vi "Get Local Framework Fields.vi"(8 "error in":errorcluster) -> (0 "error out":errorcluster, 3 "ATS Framework Fields out":T1)   [LabVIEW 2022 SP3]
uses:
  Arcadia/Common/Framework/ATS Framework Fields.ctl
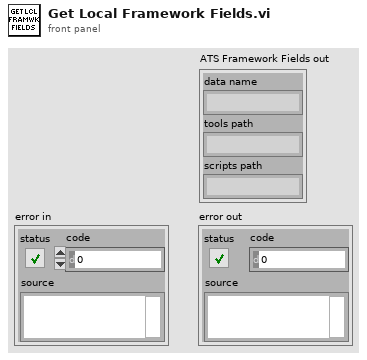
[diagram p1: front panel]
types:
  T1 = typedef "ATS Framework Fields.ctl" = cluster{"data name":string, "tools path":string, "scripts path":string}
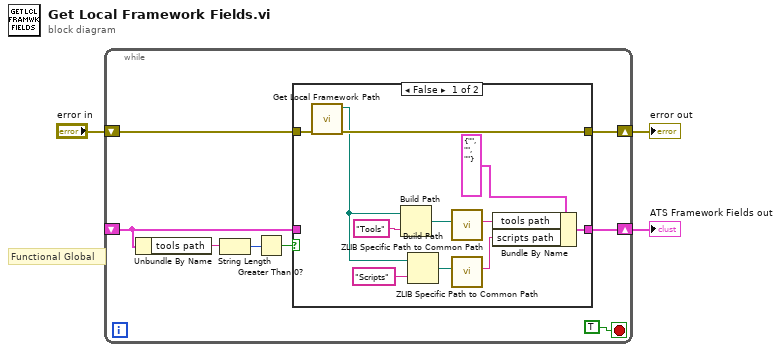
[diagram p0: block diagram]
diagram:
  # "Functional Global"
  n1 = while {
    shift-right: [w10] -> w2
    shift-left: "error in" -> [w9]
    shift-right: [w11] -> w3
    shift-left: _ -> [w4]
    stop <- TRUE stop-if-true
    n2 = Unbundle By Name(w4) -> ("tools path"=w7:string)
    n3 = String Length(string=w7) -> (length=w6:i32)
    n4 = Greater Than 0?(x=w6) -> (x > 0?=w5:bool)
    n5 = case shown="False" w5 {
      tunnel: [w22 w23] -> w11
      tunnel: [w21 w24] -> w10
      tunnel: w9 -> [w20 w24]
      tunnel: w4 -> [_ w23]
      frame False {
        n6 = call "Get Local Framework Path.vi"("error in"=w20) -> ("error out"=w21:errorcluster, "path out"=w13:path)  [unwired: 9 in]
        n7 = Build Path(base path=w13, name or relative path="Tools") -> (appended path=w16:path)
        n8 = Build Path(base path=w13, name or relative path="Scripts") -> (appended path=w17:path)
        n9 = call "ZLIB Specific Path to Common Path.vi"("specific path"=w16) -> ("common path"=w18:string)  [unwired: 10 in]
        n10 = call "ZLIB Specific Path to Common Path.vi"("specific path"=w17) -> ("common path"=w19:string)  [unwired: 10 in]
        n11 = Bundle By Name(cluster=T1 {"data name"="", "tools path"="", "scripts path"=""} ("ATS Framework Fields in"), "tools path"=w18, "scripts path"=w19) -> (w22:T1)
      }
      frame True {
      }
    }
  }
  "ATS Framework Fields out" <- w3
  "error out" <- w2
